vi "serial_08.vi"(0 "VISA resource name":refnum<visa-resource-name>="COM4") -> ()   [LabVIEW 2010]
doc: "The Basic Serial Read and Write example performs a Serial Port Read, a Serial Port Write, or a combination of these actions. The user selects the actions (read or write) on the front panel. If both are selected, the VI will write the data first, read data, and then close the VISA session that is opened to the port. This VI will wait until the specified number of bytes is received at the port. Only the number of bytes specified will be read.\n\nINSTRUCTIONS:\n1) Select the serial resource and configuration parameters (baud rate, data bits, parity, stop bits, flow control).\n2) Select the operations to be performed. \n3) Connect the serial port to your device. If no device is available, perform a loopback test by doing one of the following. Short pins 2 and 3 on a RS-232 cable or short pin 4 to pin 8 and pin 5 to pin 9 on a RS-485/422 cable. \n4) Run the VI to see the data read. (The \"read string\" will match the \"string to write\" if a loopback test was performed.)\n\nNote: The parameters set for the serial port must match the parameters of the connected instrument or device. In this example, the bytes to read parameter specifies the number of bytes that the serial port reads. If there were more bytes at the port than the number specified in bytes to read, those bytes would not be read. Also, if you specify to read more bytes than the number of bytes actually read, you might receive a timeout error message.\n\nOn the block diagram, the Configure Serial Port VI sets the configuration parameters. The front panel displays the controls used to configure the basic parameters, such as baud rate, data bits, and parity. Constants configure the other parameters the user probably does not need set. After the VISA Configure Serial Port VI opens the VISA session and configures the port, the VI passes the VISA resource name to other VIs that perform operations on that VISA resource. The VISA Write function sends a command to the serial device and the VISA Read function returns data based on the command. The VISA Close function then closes the reference to the serial device. It is important to close the reference; otherwise communication through with that port through protocols other than VISA might not be possible."
panel:
  out "Comutatoare":bool[](array[boolean])
  out "Leduri":bool[](array[boolean])
  in  "Start":bool=TRUE
  # "Stop"
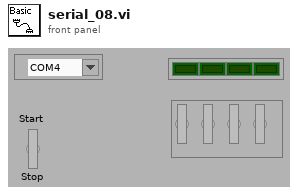
[diagram p1: front panel]
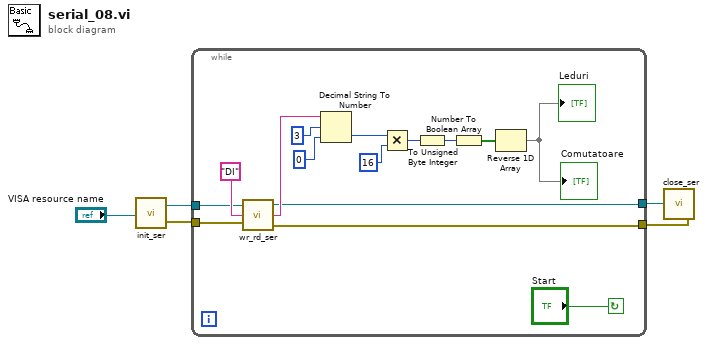
[diagram p0: block diagram]
diagram:
  n1 = call "init_ser.vi"("VISA resource name"="VISA resource name") -> ("VISA resource name out"=w3:refnum<visa-resource-name>, "error out"=w4:errorcluster)
  n2 = while {
    tunnel: w4 -> [w17]
    tunnel: w3 -> [w18]
    tunnel: [w12] -> w2
    tunnel: [w13] -> w1
    stop <- "Start" continue-if-true
    n3 = call "wr_rd_ser.vi"("error in"=w17, "string to write"="DI", "VISA resource name in"=w18) -> ("error out"=w12:errorcluster, "read buffer"=w16:string, "VISA resource name out"=w13:refnum<visa-resource-name>)
    n4 = Decimal String To Number(string=w16, offset=3, default (0L)=0) -> (number=w11:i32)  [unwired: 1 out]
    n5 = Multiply(x=w11, y=16) -> (x*y=w7:i32)
    n6 = To Unsigned Byte Integer(number=w7) -> (unsigned 8bit integer=w6:u8)
    n7 = Number To Boolean Array(number=w6) -> (Boolean array=w9:bool[])
    n8 = Reverse 1D Array(array=w9) -> (reversed array=→"Leduri" →"Comutatoare":bool[])
  }
  n9 = call "close_ser.vi"("error in"=w2, "VISA resource name in"=w1) -> ()
